vi "3458A Check Addresses.vi"(8 "error in":errorcluster, 11 "digitizer session in":T1 {"channels"."Range [Vpk]" min=0.0}) -> (0 "error out":errorcluster, 1 "some dmms shares the same controller?":bool, 2 "GPIB board numbers":u16[](array[numeric]), 3 "digitizer session out":T1 {"channels"."Range [Vpk]" min=0.0})   [LabVIEW 2018, in "3458A Virtual Digitizer.lvlib"]
doc: "3458A digitize lib: Check whether each 3458A unit has its own controller in a stream mode. It ignores input error but generates error if the condition is not meet."
uses:
  3458A Virtual Digitizer.lvlib
  3458A Digitizer Session.ctl
  3458A Virtual Channel Config.ctl
  Counter/Counter Session.ctl
  Counter/Counter Type.ctl
  AWG/AWG Session.ctl
  AWG/AWG Type.ctl
  3458A Sync Mode.ctl
  3458A Idn Mode.ctl
  3458A Digitizing Low Levels/Configure/Sampling Mode.ctl
  3458A Digitizing Process Options.ctl
  3458A Data Packet.ctl
  3458A Aux Record Data.ctl
  3458A Digitizing Low Levels/Configure/Level Setup.ctl
  3458A Digitizing Low Levels/Configure/First Sample Trigger.ctl
  3458A Aperture Selection Mode.ctl
  <vilib>/Utility/error.llb/Error Cluster From Error Code.vi
  <vilib>/regexp/Match Regular Expression.xnode
  <vilib>/ErrorRing/Error Ring.xnode
  Counter/Counter.lvlib
  AWG/AWG.lvlib
  3458A Digitizing Low Levels/3458A Digitizing Low Levels.lvlib
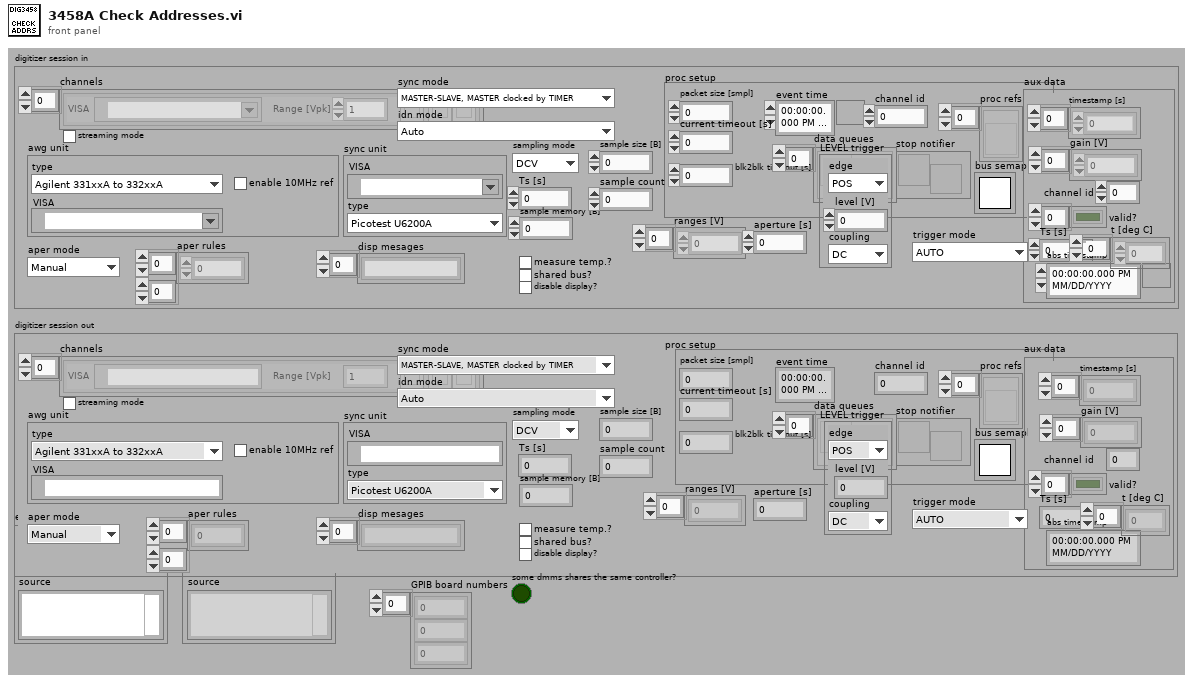
[diagram p1: front panel]
types:
  T1 = typedef "3458A Virtual Digitizer.lvlib/3458A Digitizer Session.ctl" = cluster{"channels":T2[], "sync unit":T3, "awg unit":T5, "sync mode":T7, "streaming mode":bool, "idn mode":T8, "sampling mode":T9, "Ts [s]":dbl, "sample memory [B]":i32, "proc setup":T10, "sample size [B]":i32, "sample count":i32, "aux data":T12, "ranges [V]":dbl[], "aperture [s]":dbl, "LEVEL trigger":T13, "trigger mode":T14, "measure temp.?":bool, "disp mesages":string[], "shared bus?":bool, "disable display?":bool, "aper mode":T15, "aper rules":dbl[][]}
  T2 = typedef "3458A Virtual Digitizer.lvlib/3458A Virtual Channel Config.ctl" = cluster{"VISA":refnum<visa-resource-name>, "Range [Vpk]":dbl, "btn clr":bool, "btn up":bool, "btn down":bool}
  T3 = typedef "Counter.lvlib/Counter Session.ctl" = cluster{"VISA":refnum<visa-resource-name>, "type":T4}
  T4 = typedef "Counter.lvlib/Counter Type.ctl" = enum16{"Picotest U6200A", "dummy"}
  T5 = typedef "AWG.lvlib/AWG Session.ctl" = cluster{"type":T6, "VISA":refnum<visa-resource-name>, "enable 10MHz ref":bool}
  T6 = typedef "AWG.lvlib/AWG Type.ctl" = enum16{"Agilent 331xxA to 332xxA", "Agilent 335xxA to 336xxA", "Tektronix AFG3101C", "dummy"}
  T7 = typedef "3458A Virtual Digitizer.lvlib/3458A Sync Mode.ctl" = enum16{"MASTER-SLAVE, MASTER clocked by TIMER", "MASTER-SLAVE, MASTER clocked by AWG", "ALL clocked by AWG", "MASTER-SLAVE, ALL clocked by TIMER", "ALL clocked by AWG with DFLL"}
  T8 = typedef "3458A Virtual Digitizer.lvlib/3458A Idn Mode.ctl" = enum16{"Auto", "Sequential (chn A, chn B, ...)", "From calibration string"}
  T9 = typedef "3458A Virtual Digitizer.lvlib/3458A Digitizing Low Levels.lvlib/Sampling Mode.ctl" = enum16{"DCV", "DSDC", "DSAC"}
  T10 = typedef "3458A Virtual Digitizer.lvlib/3458A Digitizing Process Options.ctl" = cluster{"channel id":i32, "packet size [smpl]":i32, "current timeout [s]":dbl, "blk2blk timeout [s]":dbl, "event time":timestamp, "stop notifier":refnum<notifier>, "data queues":refnum<queue>[], "proc refs":refnum<vi>[], "bus semaphore":T11}
  T11 = typedef "Semaphore RefNum" = refnum<k1>
  T12 = typedef "3458A Virtual Digitizer.lvlib/3458A Aux Record Data.ctl" = cluster{"channel id":i32, "valid?":bool[], "gain [V]":dbl[], "timestamp [s]":dbl[], "Ts [s]":dbl, "abs timestamp":timestamp, "t [deg C]":dbl[]}
  T13 = typedef "3458A Virtual Digitizer.lvlib/3458A Digitizing Low Levels.lvlib/Level Setup.ctl" = cluster{"edge":enum16{"POS", "NEG"}, "level [V]":dbl, "coupling":enum16{"DC", "AC"}}
  T14 = typedef "3458A Virtual Digitizer.lvlib/3458A Digitizing Low Levels.lvlib/First Sample Trigger.ctl" = enum16{"AUTO", "EXT", "SYN", "SGL", "HOLD", "LEVEL"}
  T15 = typedef "3458A Virtual Digitizer.lvlib/3458A Aperture Selection Mode.ctl" = enum16{"Manual", "Maximum", "Table"}
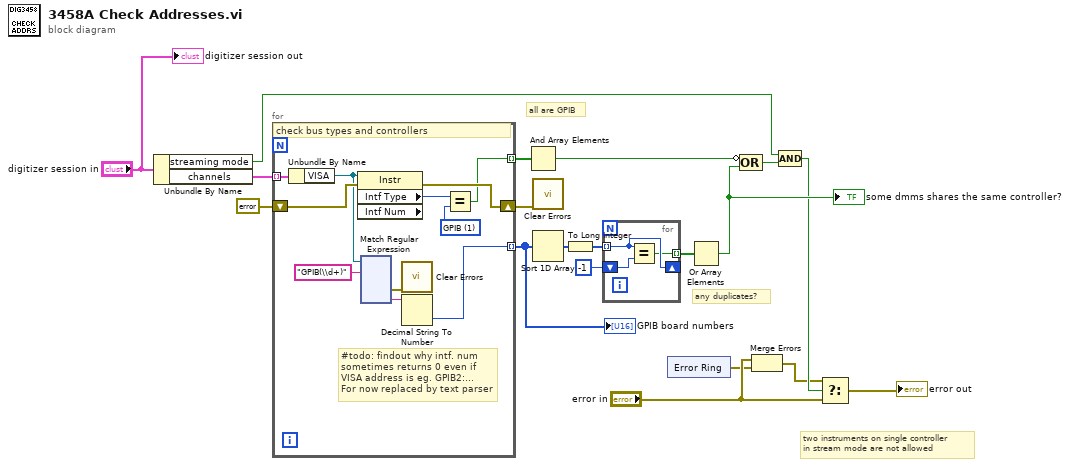
[diagram p0: block diagram]
diagram:
  # "two instruments on single controller\nin stream mode are not allowed"
  # "any duplicates?"
  # "all are GPIB"
  n1 = Unbundle By Name("digitizer session in") -> ("streaming mode"=w7:bool, "channels"=w18:T2[])
  n2 = for {
    tunnel: w18 -> [w30] mode=indexing
    shift-right: [w26] -> w11
    shift-left: errorcluster {"status"=FALSE, "code"=0, "source"=""} ("error out") -> [w29]
    tunnel: [w20] -> w16 mode=indexing
    tunnel: [w25] -> w17 mode=indexing
    w27 = u16 1 items=["GPIB"=1, "VXI"=2, "GPIB-VXI"=3, "Serial"=4, "PXI"=5, "TCPIP"=6, "USB"=7, "FireWire"=9] ("Interface Information:Interface Type")
    # "#todo: findout why intf. num\nsometimes returns 0 even if \nVISA address is eg. GPIB2:...\nFor now replaced by text parser"
    # "check bus types and controllers"
    n3 = Unbundle By Name(w30) -> ("VISA"=w24:refnum<visa-resource-name>)
    n4 = property class="Instr" props=["Intf Type", "Intf Num"](reference=w24, error in=w29) -> (error out=w26:errorcluster, "Intf Type"=w28:u16)  [unwired: 2 out]
    n5 = xnode "Match Regular Expression"("input string"=w24, "regular expression"="GPIB(\\d+)") -> ("error out"=w21:errorcluster, "submatch 1"=w22:string)  [unwired: 4 in, 4 out]
    n6 = call <vilib>:"Clear Errors.vi"("error in (no error)"=w21) -> ()  [unwired: 5 in, 2 out]
    n7 = Decimal String To Number(string=w22) -> (number=w20:i32)  [unwired: 2 in, 1 out]
    n8 = Equal?(x=w28, y=w27) -> (x = y?=w25:bool)
  }
  "GPIB board numbers" <- w16
  n9 = And Array Elements(Boolean array=w17) -> (logical AND=w10:bool)
  n10 = call <vilib>:"Clear Errors.vi"("error in (no error)"=w11) -> ()  [unwired: 5 in, 2 out]
  n11 = Sort 1D Array(array=w16) -> (sorted array=w15:i32[])
  n12 = To Long Integer(number=w15) -> (32bit integer=w13:i32[])
  n13 = for {
    tunnel: w13 -> [w148] mode=indexing
    shift-right: [w148] -> _
    shift-left: -1 -> [w149]
    tunnel: [w147] -> w12 mode=indexing
    n14 = Equal?(x=w148, y=w149) -> (x = y?=w147:bool)
  }
  n15 = xnode "Error Ring"() -> ("error out"=w2:errorcluster)
  n16 = Or Array Elements(Boolean array=w12) -> (logical OR=w9:bool)
  "some dmms shares the same controller?" <- w9
  n17 = Compound Arithmetic op=OR(invert w10, w9) -> (w8:bool)
  n18 = Merge Errors("error in", w2) -> (w3:errorcluster)
  n19 = Compound Arithmetic op=AND(w7, w8) -> (w6:bool)
  n20 = Select(t=w3, s=w6, f="error in") -> (s? t:f=→"error out":errorcluster)
  "digitizer session out" <- "digitizer session in"
